vi "control_pane_ui_handler.vi"(8 "error in (no error)":errorcluster, 11 "Control Panel In":refnum<vi>) -> (0 "error out":errorcluster)   [LabVIEW 2019]
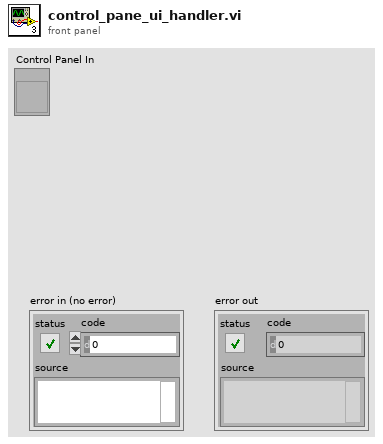
[diagram p1: front panel]
types:
  T1 = enum8{"Enabled", "Disabled", "Disabled and Grayed Out"}
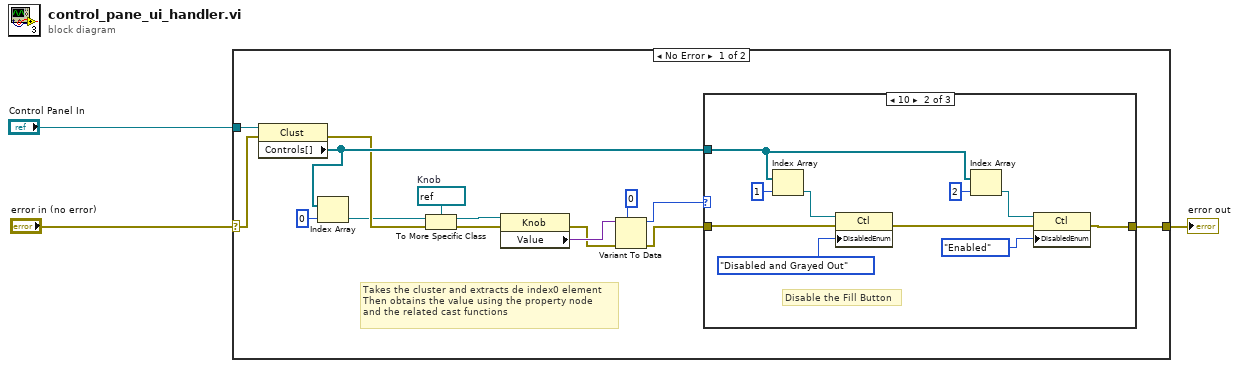
[diagram p0: block diagram]
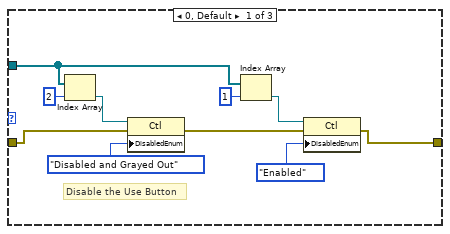
[diagram p2: hidden frame]
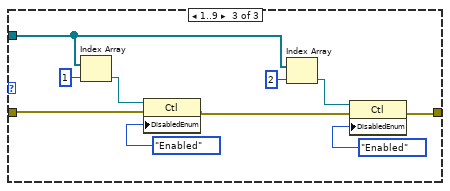
[diagram p3: hidden frame]
diagram:
  n1 = case shown="No Error" "error in (no error)" {
    selector: "error in (no error)" -> [w16 w49]
    tunnel: [w18 w49] -> w2
    tunnel: "Control Panel In" -> [w17 _]
    frame No Error {
      w9 = refnum<vi> refnum  # Knob
      # "Takes the cluster and extracts de index0 element\nThen obtains the value using the property node \nand the related cast functions"
      n2 = property class="Clust"(reference=w17, error in=w16) -> (error out=w13:errorcluster, "Controls[]"=w14:refnum<vi>[])  [unwired: 1 out]
      n3 = Index Array(array=w14, index=0) -> (element=w12:refnum<vi>)
      n4 = To More Specific Class(target class=w9, reference=w12, error in=w13) -> (specific class reference=w11:refnum<vi>, error out=w10:errorcluster)
      n5 = property class="Knob"(reference=w11, error in=w10) -> (error out=w6:errorcluster, "Value"=w8:variant)  [unwired: 1 out]
      n6 = Variant To Data(error in=w6, type=i8 0 ("Value"), Variant=w8) -> (data=w4:i8, error out=w5:errorcluster)
      n7 = case shown="10" w4 {
        tunnel: [w23 w30 w39] -> w18
        tunnel: w14 -> [w21 w29 w41]
        tunnel: w5 -> [w27 w35 w45]
        frame 0, Default {
          # "Disable the Use Button"
          n8 = Index Array(array=w21, index=2) -> (element=w25:refnum<vi>)
          n9 = property class="Ctl"(reference=w25, error in=w27, "DisabledEnum"=T1."Disabled and Grayed Out" ("Disabled")) -> (error out=w22:errorcluster)  [unwired: 1 out]
          n10 = Index Array(array=w21, index=1) -> (element=w24:refnum<vi>)
          n11 = property class="Ctl"(reference=w24, error in=w22, "DisabledEnum"=T1."Enabled" ("Disabled")) -> (error out=w23:errorcluster)  [unwired: 1 out]
        }
        frame 10 {
          # "Disable the Fill Button"
          n12 = Index Array(array=w29, index=1) -> (element=w36:refnum<vi>)
          n13 = property class="Ctl"(reference=w36, error in=w35, "DisabledEnum"=T1."Disabled and Grayed Out" ("Disabled")) -> (error out=w31:errorcluster)  [unwired: 1 out]
          n14 = Index Array(array=w29, index=2) -> (element=w34:refnum<vi>)
          n15 = property class="Ctl"(reference=w34, error in=w31, "DisabledEnum"=T1."Enabled" ("Disabled")) -> (error out=w30:errorcluster)  [unwired: 1 out]
        }
        frame 1..9 {
          n16 = Index Array(array=w41, index=1) -> (element=w46:refnum<vi>)
          n17 = property class="Ctl"(reference=w46, error in=w45, "DisabledEnum"=T1."Enabled" ("Disabled")) -> (error out=w40:errorcluster)  [unwired: 1 out]
          n18 = Index Array(array=w41, index=2) -> (element=w44:refnum<vi>)
          n19 = property class="Ctl"(reference=w44, error in=w40, "DisabledEnum"=T1."Enabled" ("Disabled")) -> (error out=w39:errorcluster)  [unwired: 1 out]
        }
      }
    }
    frame Error {
    }
  }
  "error out" <- w2
